vi "initialise_keithley_j-t.vi"(10 "J-t Scan Settings":T1={"Bias 1"=20.0, "Bias 2 "=0.0, "t for bias 1 (s)"=60.0, "t for bias 2 (s)"=120.0, "Enable display"=0, "Electrode configuration"=0, "Bias 1 mode"=0, "Bias 2 mode"=0, "Current range for bias 1"=0, "Current range for bias 2"=0, "Voltage range for bias 1"=0, "Voltage range for bias 2"=0, "Settling delay (ms)"=1.0, "Auto settling delay"=1, "Integration time (ms)"=1.0} {"Integration time (ms)" min=0.2; "Auto settling delay" items=["False", "True"]; "Settling delay (ms)" min=0.0; "Voltage range for bias 2" items=["Auto", "200 mV", "2 V", "20 V", "200 V"]; "Voltage range for bias 1" items=["Auto", "200 mV", "2 V", "20 V", "200 V"]; "Current range for bias 2" items=["Auto", "1 uA", "10 uA", "100 uA", "1 mA", "10 mA", "100 mA", "1 A"]; "Current range for bias 1" items=["Auto", "1 uA", "10 uA", "100 uA", "1 mA", "10 mA", "100 mA", "1 A"]; "Bias 2 mode" items=["V", "A"]; "Bias 1 mode" items=["V", "A"]; "Electrode configuration" items=["2-wire", "4-wire"]; "Enable display" items=["False", "True"]; "t for bias 2 (s)" min=0.0; "t for bias 1 (s)" min=0.0}, 11 "VISA Refnum in":refnum<visa-resource-name>="GPIB1::26::INSTR") -> (0 "error out":errorcluster, 3 "VISA Refnum out":refnum<visa-resource-name>)   [LabVIEW 2016]
uses:
  TypeDefs/j-t_settings.ctl
  <instrlib>/Keithley 24XX/Keithley 24XX.lvlib
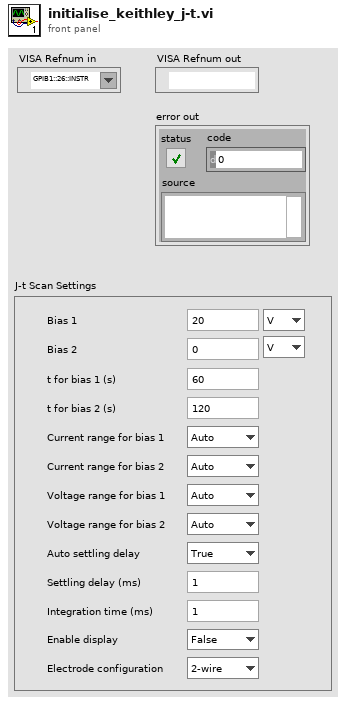
[diagram p1: front panel]
types:
  T1 = typedef "j-t_settings.ctl" = cluster{"Bias 1":dbl, "Bias 2 ":dbl, "t for bias 1 (s)":dbl, "t for bias 2 (s)":dbl, "Enable display":u16, "Electrode configuration":u16, "Bias 1 mode":u16, "Bias 2 mode":u16, "Current range for bias 1":u16, "Current range for bias 2":u16, "Voltage range for bias 1":u16, "Voltage range for bias 2":u16, "Settling delay (ms)":dbl, "Auto settling delay":u16, "Integration time (ms)":dbl}
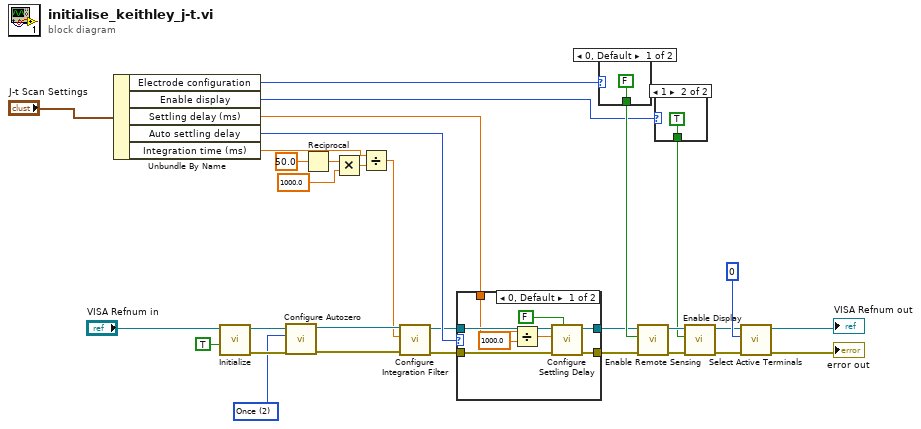
[diagram p0: block diagram]
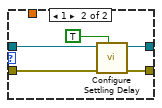
[diagram p2: hidden frame]
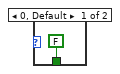
[diagram p3: hidden frame]
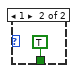
[diagram p4: hidden frame]
diagram:
  w20 = u16 2 items=["On", "Off", "Once"] ("Autozero  (0: On)")
  n1 = Unbundle By Name("J-t Scan Settings") -> ("Electrode configuration"=w19:u16, "Enable display"=w14:u16, "Settling delay (ms)"=w6:dbl, "Auto settling delay"=w5:u16, "Integration time (ms)"=w7:dbl)
  n2 = call <instrlib>:"Initialize.vi"("Reset (True)"=TRUE, "VISA resource name"="VISA Refnum in") -> ("error out"=w21:errorcluster, "VISA resource name out"=w22:refnum<visa-resource-name>)  [unwired: 3 in, 5 out]
  n3 = call <instrlib>:"Configure Autozero.vi"("error in (no error)"=w21, "Autozero  (0: On)"=w20, "VISA resource name"=w22) -> ("error out"=w15:errorcluster, "VISA resource name out"=w16:refnum<visa-resource-name>)  [unwired: 7 in]
  n4 = Reciprocal(x=50.0) -> (1/x=w11:dbl)
  n5 = Multiply(x=w11, y=1000.0) -> (x*y=w9:dbl)
  n6 = Divide(x=w7, y=w9) -> (x/y=w8:dbl)
  n7 = call <instrlib>:"Configure Integration Filter.vi"("error in (no error)"=w15, "Measurement Speed (1 PLC)"=w8, "VISA resource name"=w16) -> ("error out"=w3:errorcluster, "VISA resource name out"=w4:refnum<visa-resource-name>)  [unwired: 7 in]
  n8 = case shown="0, Default" w5 {
    tunnel: [w39 w44] -> w2
    tunnel: [w38 w43] -> w1
    tunnel: w4 -> [w37 w41]
    tunnel: w3 -> [w36 w42]
    tunnel: w6 -> [w34 _]
    frame 0, Default {
      n9 = Divide(x=w34, y=1000.0) -> (x/y=w35:dbl)
      n10 = call <instrlib>:"Configure Settling Delay.vi"("Auto Settle (T: Enable)"=FALSE, "error in (no error)"=w36, "Manual Settling Delay (0 sec)"=w35, "VISA resource name"=w37) -> ("error out"=w38:errorcluster, "VISA resource name out"=w39:refnum<visa-resource-name>)  [unwired: 6 in]
    }
    frame 1 {
      n11 = call <instrlib>:"Configure Settling Delay.vi"("Auto Settle (T: Enable)"=TRUE, "error in (no error)"=w42, "VISA resource name"=w41) -> ("error out"=w43:errorcluster, "VISA resource name out"=w44:refnum<visa-resource-name>)  [unwired: 7 in]
    }
  }
  n12 = case shown="0, Default" w19 {
    tunnel: [FALSE ("Enable Output (T: Enable)") TRUE ("Enable Output (T: Enable)")] -> w18
    frame 0, Default {
    }
    frame 1 {
    }
  }
  n13 = call <instrlib>:"Enable Remote Sensing.vi"("error in (no error)"=w1, "Enable Remote Sensing (T: Enable)"=w18, "VISA resource name"=w2) -> ("error out"=w25:errorcluster, "VISA resource name out"=w24:refnum<visa-resource-name>)  [unwired: 7 in]
  n14 = case shown="1" w14 {
    tunnel: [FALSE ("Enable Output (T: Enable)") TRUE ("Enable Output (T: Enable)")] -> w13
    frame 0, Default {
    }
    frame 1 {
    }
  }
  n15 = call <instrlib>:"Enable Display.vi"("error in (no error)"=w25, "Enable Display (T: Enable)"=w13, "VISA resource name"=w24) -> ("error out"=w27:errorcluster, "VISA resource name out"=w26:refnum<visa-resource-name>)  [unwired: 7 in]
  n16 = call <instrlib>:"Select Active Terminals.vi"("error in (no error)"=w27, "Active Terminals (0: Front)"=0, "VISA resource name"=w26) -> ("error out"=→"error out":errorcluster, "VISA resource name out"=→"VISA Refnum out":refnum<visa-resource-name>)  [unwired: 7 in]
